vi "ClassLoader_lib.vi"() -> (0 "ClassLoader_lib":refnum<class "ClassLoader_lib.lvclass">)   [LabVIEW 2020, in "ClassLoader_VIMs.lvlib"]
uses:
  ClassLoader_VIMs.lvlib
  ClassLoader_lib/ClassLoader_lib.lvclass
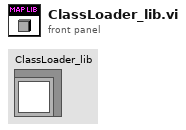
[diagram p1: front panel]
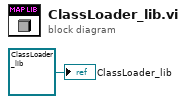
[diagram p0: block diagram]
diagram:
  "ClassLoader_lib" <- refnum<class "ClassLoader_lib.lvclass"> refnum ("ClassLoader.lvlib:ClassLoader_lib.lvclass")
